vi "PSDEV_Device Run ConfigEXE.vi"(8 "error in":errorcluster caption="错误输入（无错误）") -> (0 "error out":errorcluster caption="错误输出")   [LabVIEW 2016]
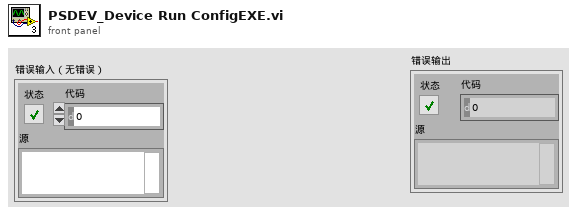
[diagram p1: front panel]
types:
  T1 = cluster{"TREE PNG":path, "User Guide":path, "DefaultSave":path, "BuildPath":path, "Image":path, "Modules":path, "Configuration":path, "License":path, "SplitFiles":path, "System.ini":path}
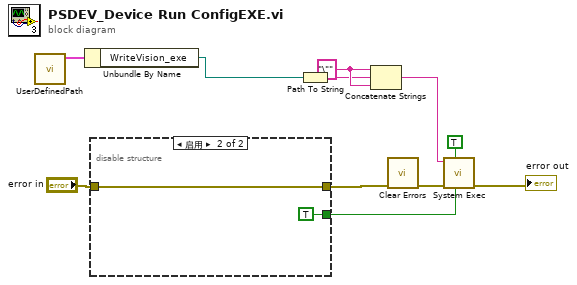
[diagram p0: block diagram]
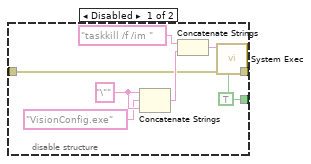
[diagram p2: hidden frame]
diagram:
  w8 = "\"" ("String")
  n1 = call "UserDefinedPath.vi"() -> ("UserDefinedPath"=w2:T1)  [unwired: 11 in]
  n2 = Unbundle By Name(w2) -> ("WriteVision_exe"=w1:path)
  n3 = disable-structure shown="启用" {
    disable-tunnel: [w19 w21] -> w6
    disable-tunnel: [w16 TRUE ("run minimized? (F)")] -> w5
    disable-tunnel: "error in" -> [w12 w21]
    frame Disabled {
      w15 = "\"" ("String")
      w16 = TRUE ("run minimized? (F)")
      n4 = Concatenate Strings(w15, "VisionConfig.exe" ("name or relative path"), w15) -> (w14:string)
      n5 = Concatenate Strings("taskkill /f /im " ("command line"), w14) -> (w18:string)
      n6 = call <vilib>:"System Exec.vi"("run minimized? (F)"=w16, "error in (no error)"=w12, "command line"=w18) -> ("error out"=w19:errorcluster)  [unwired: 5 in, 3 out]
    }
    frame Enabled {
    }
  }
  n7 = Path To String(path=w1) -> (string=w7:string)
  n8 = Concatenate Strings(w8, w7, w8) -> (w9:string)
  n9 = call <vilib>:"Clear Errors.vi"("error in (no error)"=w6) -> ("error out"=w10:errorcluster)  [unwired: 5 in, 1 out]
  n10 = call <vilib>:"System Exec.vi"("run minimized? (F)"=w5, "wait until completion? (T)"=TRUE, "error in (no error)"=w10, "command line"=w9) -> ("error out"=→"error out":errorcluster)  [unwired: 4 in, 3 out]
